vi "Toggle Draw Lines.vi"(11 "Scene in":refnum<class "Scene.lvclass">) -> (3 "Scene out":refnum<class "Scene.lvclass">)   [LabVIEW 2020, in "Application.lvlib" / "Scene.lvclass"]
uses:
  Scene.lvclass
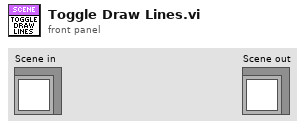
[diagram p1: front panel]
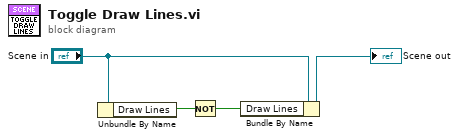
[diagram p0: block diagram]
diagram:
  n1 = Unbundle By Name("Scene in") -> ("Draw Lines"=w2:bool)
  n2 = Not(x=w2) -> (.not. x?=w1:bool)
  n3 = Bundle By Name(cluster="Scene in", "Draw Lines"=w1) -> (→"Scene out":refnum<class "Scene.lvclass">)
